vi "Reporte.vi"() -> ()   [LabVIEW 2026]
uses:
  <vilib>/Utility/NIReport.llb/NI_report.lvclass
  <vilib>/Utility/NIReport.llb/Report Type.ctl
  <vilib>/Utility/NIReport.llb/NI_ReportGenerationCore.lvlib
  <vilib>/Utility/NIReport.llb/image depth.ctl
  <vilib>/printing/OpenHTMLReport.llb/Open HTML Report in Browser (Refnum).vi
panel:
  in  "Knob":dbl(knob) scale=0.0..10.0
  out "Waveform Chart":dbl(graph)
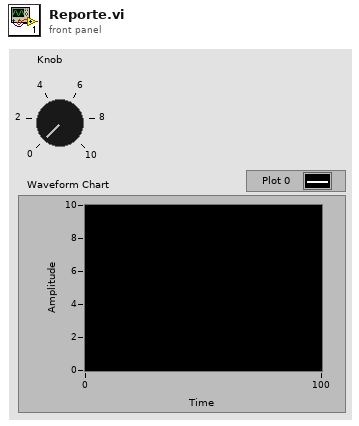
[diagram p1: front panel]
types:
  T1 = typedef "NI_ReportGenerationCore.lvlib/image depth.ctl" = u16
  T2 = typedef "NI_ReportGenerationCore.lvlib/Report Type.ctl" = enum16{"HTML", "Word", "Excel"}
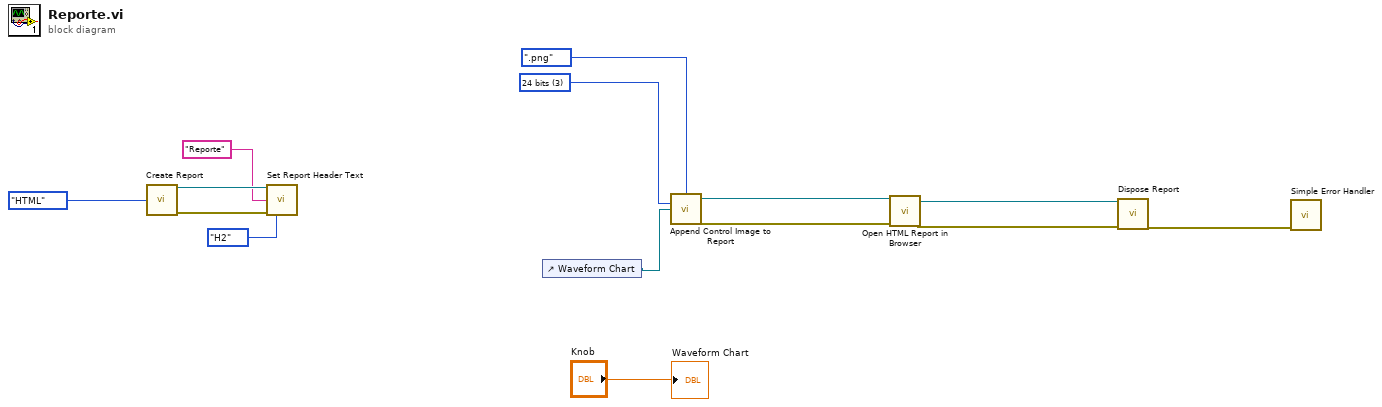
[diagram p0: block diagram]
diagram:
  w8 = T1 3 items=["B&W", "4 bits", "8 bits", "24 bits"] ("image depth")
  n1 = call <vilib>:"Create Report.vi"("report type"=Report_Type."HTML") -> ("report out"=w13:refnum<class "NI_report.lvclass">, "error out"=w12:errorcluster)  [unwired: 13 in]
  n2 = call-dynamic "Set Report Header Text.vi"("report in"=w13, "center header text"="Reporte", "error in (no error)"=w12, "HTML header size"=enum16{"H1", "H2", "H3", "H4", "H5", "H6", "H7"}."H2") -> ()  [unwired: 10 in, 2 out]
  n3 = control-ref of="Waveform Chart"() -> (w7:refnum<vi>)
  n4 = call-dynamic "Append Control Image to Report.vi"("image file type (.jpg)"=enum16{".jpg", ".png"}.".png", "image depth"=w8, "ctrl reference"=w7) -> ("report out"=w6:refnum<class "NI_report.lvclass">, "error out"=w5:errorcluster)  [unwired: 9 in, 2 out]
  n5 = call-poly <vilib>:"Open HTML Report in Browser.vi"("report in"=w6, "error in (no error)"=w5) -> ("report out"=w4:refnum<class "NI_report.lvclass">, "error out"=w3:errorcluster)  [unwired: 11 in, 1 out]
  n6 = call-dynamic "Dispose Report.vi"("report in"=w4, "error in (no error)"=w3) -> ("error out"=w2:errorcluster)  [unwired: 13 in]
  n7 = call <vilib>:"Simple Error Handler.vi"("error in (no error)"=w2) -> ()  [unwired: 4 in, 5 out]
  "Waveform Chart" <- "Knob"
